vi "2048_check_removable.vi"(10 "Array in":i32[][](array[numeric]), 11 "Numeric in":i32) -> (2 "isremovable":bool, 3 "Numeric out":i32)   [LabVIEW 2022 SP3]
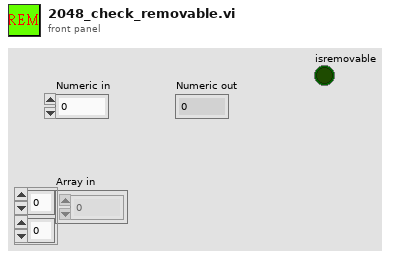
[diagram p1: front panel]
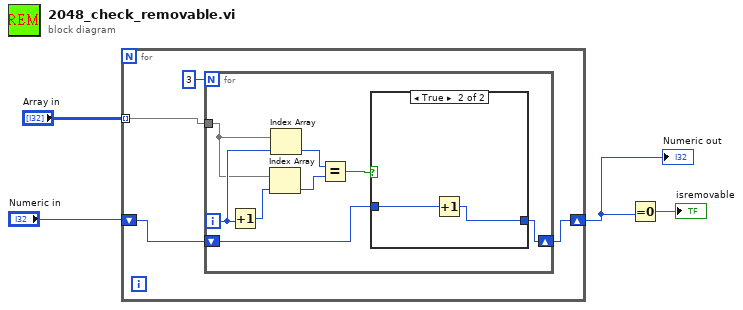
[diagram p0: block diagram]
diagram:
  n1 = for {
    tunnel: "Array in" -> [w7] mode=indexing
    shift-right: [w5] -> w2
    shift-left: "Numeric in" -> [w6]
    n2 = for {
      N: 3 -> [_]
      tunnel: w7 -> [w11]
      shift-right: [w9] -> w5
      shift-left: w6 -> [w10]
      i -> [w16]
      n3 = Increment(x=w16) -> (x+1=w15:i32)
      n4 = Index Array(array=w11, index=w15) -> (element=w14:i32)
      n5 = Index Array(array=w11, index=w16) -> (element=w13:i32)
      n6 = Equal?(x=w13, y=w14) -> (x = y?=w12:bool)
      n7 = case shown="True" w12 {
        tunnel: w10 -> [w17 w19]
        tunnel: [w17 w18] -> w9
        frame False {
        }
        frame True {
          n8 = Increment(x=w19) -> (x+1=w18:i32)
        }
      }
    }
  }
  "Numeric out" <- w2
  n9 = Equal To 0?(x=w2) -> (x = 0?=→"isremovable":bool)
